vi "Configure Air Flow Setpoint in scfm.vi"(8 "error in (no error)":errorcluster, 9 "Air Flow Setpoint (12)":dbl=12.0 min=0.0 max=25.0 step=1.0, 11 "VISA resource name":refnum<visa-resource-name>) -> (0 "error out":errorcluster, 3 "VISA resource name out":refnum<visa-resource-name>)   [LabVIEW 2010, in "Temptronic TP04300.lvlib"]
doc: "This VI configures air flow setpoint in scfm for TP04300 instrument.\n<b>Air Flow Setpoint, in scfm</b> - used to configure the main nozzle air flow \nrate in scfm.\n\nDefault Value: 12 \nValid Range: 2 - 18"
uses:
  Temptronic TP04300.lvlib
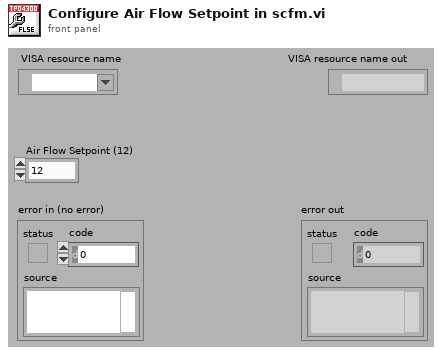
[diagram p1: front panel]
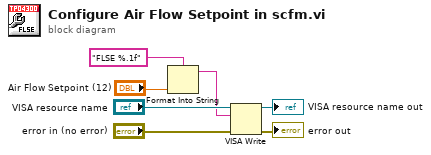
[diagram p0: block diagram]
diagram:
  n1 = Format Into String(format string="FLSE %.1f" ("multi-line string"), "Air Flow Setpoint (12)") -> (resulting string=w3:string)  [unwired: 2 in, 1 out]
  n2 = VISA Write(VISA resource name="VISA resource name", write buffer=w3, error in (no error)="error in (no error)") -> (VISA resource name out=→"VISA resource name out":refnum<visa-resource-name>, error out=→"error out":errorcluster)  [unwired: 1 out]
